vi "Read Dates.vi"(7 "SN":T2, 8 "error in (no error)":errorcluster, 9 "Calibration ID":T1, 10 "Time Stamp in":T3 {"Chamber Temp" format="%<%x>T"; "Probe 2 Temp" format="%<%x>T"; "Probe 1 Temp" format="%<%x>T"; "TC Panel 2" format="%<%x>T"; "TC Panel 1" format="%<%x>T"; "NI DAQ Card 7" format="%<%x>T"; "NI DAQ Card 6" format="%<%x>T"; "NI DAQ Card 5" format="%<%x>T"; "NI DAQ Card 4" format="%<%x>T"; "NI DAQ Card 3" format="%<%x>T"; "NI DAQ Card 2" format="%<%x>T"; "NI DAQ Card 1" format="%<%x>T"; "Gas Meter Thermocouple" format="%<%x>T"; "Gas Meter Pressure Transducer" format="%<%x>T"; "Gas Meter" format="%<%x>T"; "Sentra Scale" format="%<%x>T"; "B-Tech Scale" format="%<%x>T"; "Barometer" format="%<%x>T"; "WT 500" format="%<%x>T"; "Chroma" format="%<%x>T"}, 11 "file path (dialog if empty)":path) -> (0 "error out":errorcluster, 1 "SN.":T2, 2 "Calibration ID.":T1, 3 "Time Stamp out":T3 {"Chamber Temp" format="%<%x>T"; "Probe 2 Temp" format="%<%x>T"; "Probe 1 Temp" format="%<%x>T"; "TC Panel 2" format="%<%x>T"; "TC Panel 1" format="%<%x>T"; "NI DAQ Card 7" format="%<%x>T"; "NI DAQ Card 6" format="%<%x>T"; "NI DAQ Card 5" format="%<%x>T"; "NI DAQ Card 4" format="%<%x>T"; "NI DAQ Card 3" format="%<%x>T"; "NI DAQ Card 2" format="%<%x>T"; "NI DAQ Card 1" format="%<%x>T"; "Gas Meter Thermocouple" format="%<%x>T"; "Gas Meter Pressure Transducer" format="%<%x>T"; "Gas Meter" format="%<%x>T"; "Sentra Scale" format="%<%x>T"; "B-Tech Scale" format="%<%x>T"; "Barometer" format="%<%x>T"; "WT 500" format="%<%x>T"; "Chroma" format="%<%x>T"}, 4 "Size":i32, 5 "new file path (Not A Path if cancelled)":path)   [LabVIEW 2014]
uses:
  Type Definitions/CalibrationTime.ctl
  Type Definitions/Calibration.ctl
  Type Definitions/Calibration_SN.ctl
  <vilib>/Utility/file.llb/Read From Spreadsheet File (string).vi
panel:
  out "all rows":string[][](array[string])
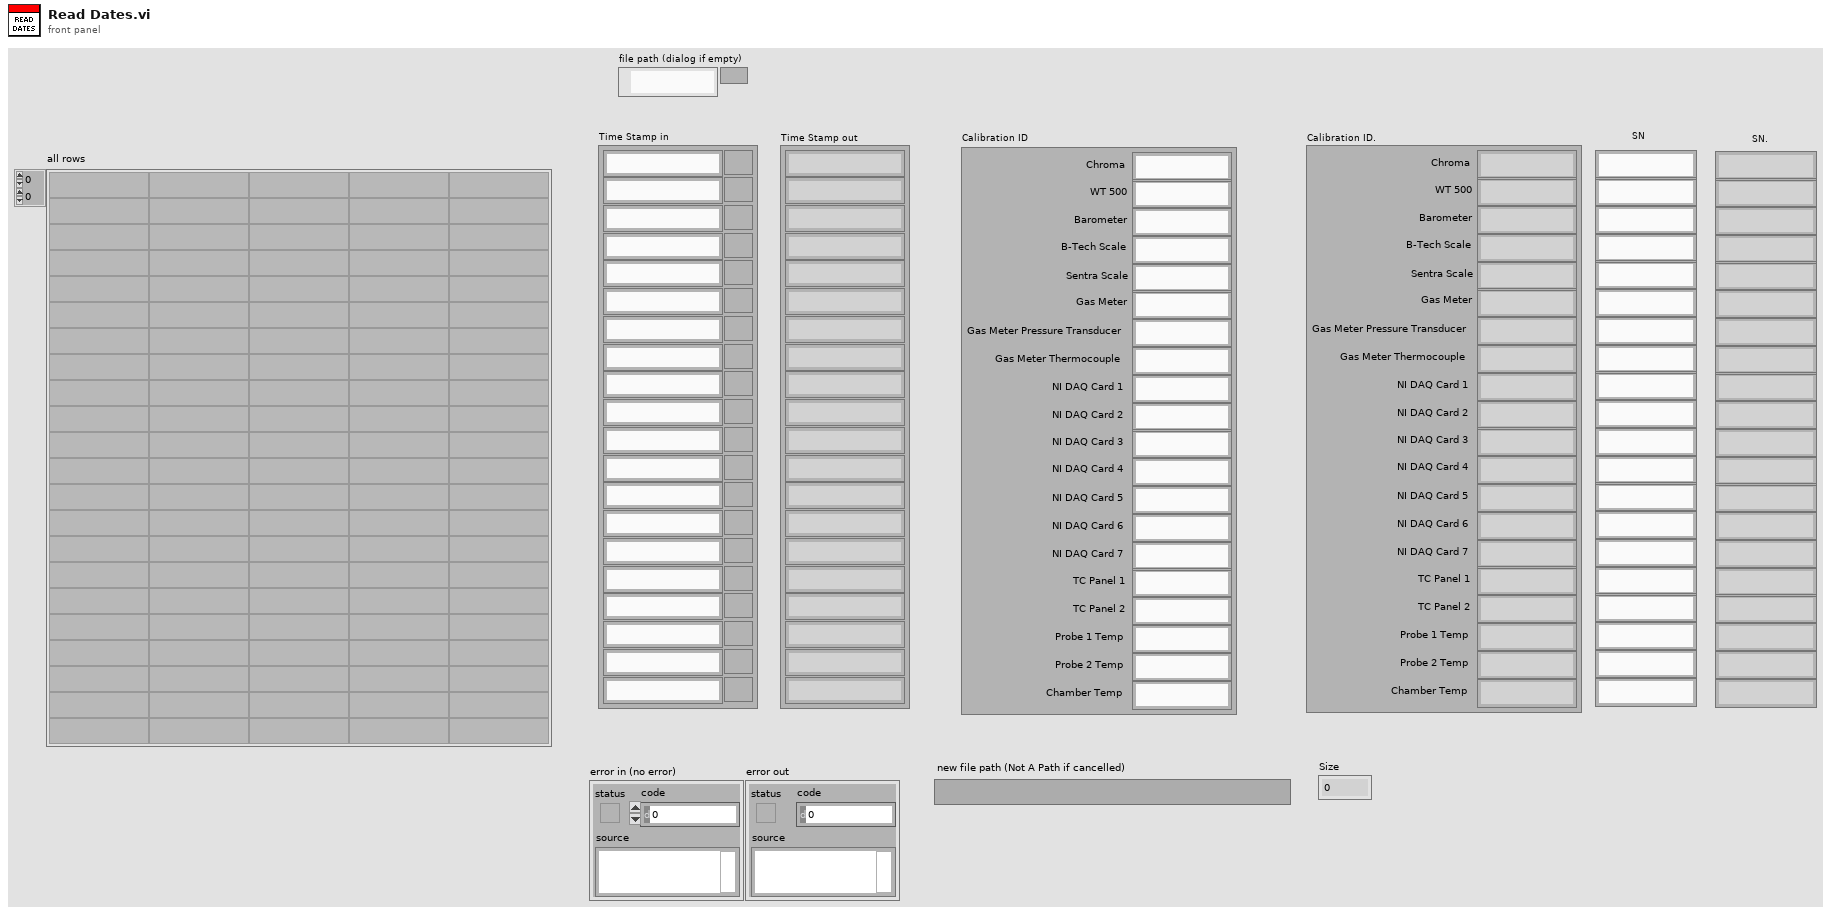
[diagram p1: front panel]
types:
  T1 = typedef "Calibration.ctl" = cluster{"Chroma":string, "WT 500":string, "Barometer":string, "B-Tech Scale":string, "Sentra Scale":string, "Gas Meter":string, "Gas Meter Pressure Transducer":string, "Gas Meter Thermocouple":string, "NI DAQ Card 1":string, "NI DAQ Card 2":string, "NI DAQ Card 3":string, "NI DAQ Card 4":string, "NI DAQ Card 5":string, "NI DAQ Card 6":string, "NI DAQ Card 7":string, "TC Panel 1":string, "TC Panel 2":string, "Probe 1 Temp":string, "Probe 2 Temp":string, "Chamber Temp":string}
  T2 = typedef "Calibration_SN.ctl" = cluster{"Chroma":string, "WT 500":string, "Barometer":string, "B-Tech Scale":string, "Sentra Scale":string, "Gas Meter":string, "Gas Meter Pressure Transducer":string, "Gas Meter Thermocouple":string, "NI DAQ Card 1":string, "NI DAQ Card 2":string, "NI DAQ Card 3":string, "NI DAQ Card 4":string, "NI DAQ Card 5":string, "NI DAQ Card 6":string, "NI DAQ Card 7":string, "TC Panel 1":string, "TC Panel 2":string, "Probe 1 Temp":string, "Probe 2 Temp":string, "Chamber Temp":string}
  T3 = typedef "CalibrationTime.ctl" = cluster{"Chroma":timestamp, "WT 500":timestamp, "Barometer":timestamp, "B-Tech Scale":timestamp, "Sentra Scale":timestamp, "Gas Meter":timestamp, "Gas Meter Pressure Transducer":timestamp, "Gas Meter Thermocouple":timestamp, "NI DAQ Card 1":timestamp, "NI DAQ Card 2":timestamp, "NI DAQ Card 3":timestamp, "NI DAQ Card 4":timestamp, "NI DAQ Card 5":timestamp, "NI DAQ Card 6":timestamp, "NI DAQ Card 7":timestamp, "TC Panel 1":timestamp, "TC Panel 2":timestamp, "Probe 1 Temp":timestamp, "Probe 2 Temp":timestamp, "Chamber Temp":timestamp}
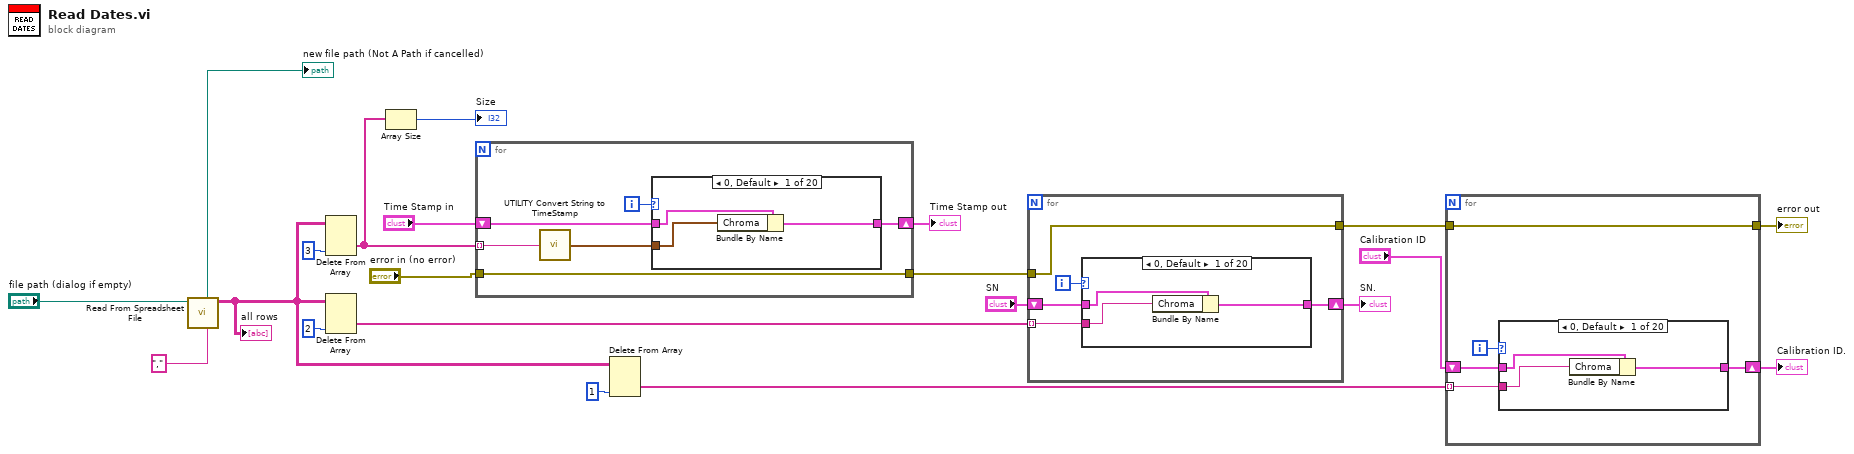
[diagram p0: block diagram]
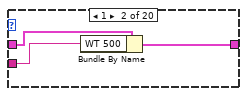
[diagram p2: hidden frame]
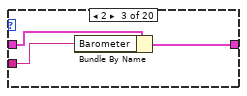
[diagram p3: hidden frame]
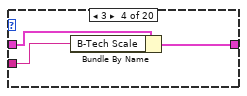
[diagram p4: hidden frame]
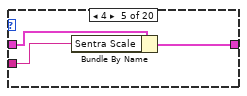
[diagram p5: hidden frame]
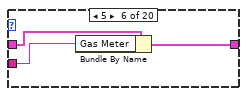
[diagram p6: hidden frame]
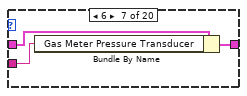
[diagram p7: hidden frame]
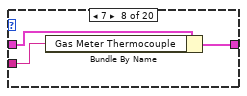
[diagram p8: hidden frame]
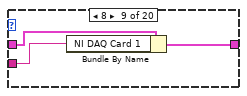
[diagram p9: hidden frame]
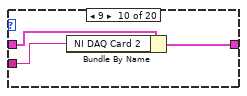
[diagram p10: hidden frame]
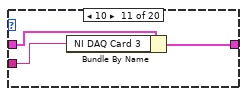
[diagram p11: hidden frame]
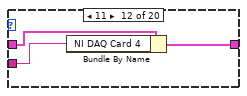
[diagram p12: hidden frame]
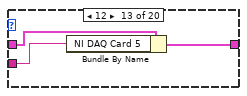
[diagram p13: hidden frame]
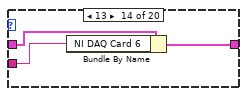
[diagram p14: hidden frame]
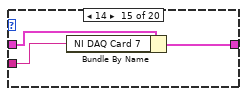
[diagram p15: hidden frame]
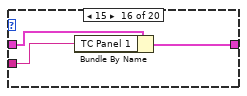
[diagram p16: hidden frame]
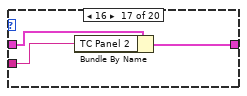
[diagram p17: hidden frame]
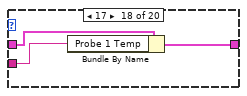
[diagram p18: hidden frame]
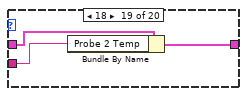
[diagram p19: hidden frame]
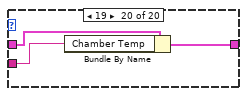
[diagram p20: hidden frame]
diagram:
  n1 = call-poly <vilib>:"Read From Spreadsheet File.vi"("delimiter (\\t)"="," ("delimiter (\\t)"), "file path (dialog if empty)"="file path (dialog if empty)") -> ("all rows"=w11:string[][], "new file path (Not A Path if cancelled)"=→"new file path (Not A Path if cancelled)":path)  [unwired: 5 in, 3 out]
  "all rows" <- w11
  n2 = Delete From Array(array=w11, index (col)=3 ("disabled index (col)")) -> (deleted portion=w2:string[])  [unwired: 2 in, 1 out]
  n3 = Delete From Array(array=w11, index (col)=2 ("disabled index (col)")) -> (deleted portion=w8:string[])  [unwired: 2 in, 1 out]
  n4 = Array Size(array=w2) -> (size(s)=→"Size":i32)
  n5 = for {
    tunnel: w2 -> [w27] mode=indexing
    shift-right: [w23] -> w18
    shift-left: "Time Stamp in" -> [w25]
    tunnel: [w22] -> w15
    tunnel: "error in (no error)" -> [w22]
    i -> [w26]
    n6 = call "UTILITY Convert String to TimeStamp.vi"("date/time string"=w27) -> ("Resulting Time Stamp"=w24:timestamp)
    n7 = case shown="0, Default" w26 {
      tunnel: w25 -> [w29 w32 w35 w38 w41 w44 w47 w50 w53 w56 w59 w62 w65 w68 w72 w75 w78 w81 w83 w86]
      tunnel: w24 -> [w30 w33 w36 w39 w42 w45 w48 w51 w54 w57 w60 w63 w66 w69 w71 w74 w77 w79 w84 w87]
      tunnel: [w28 w31 w34 w37 w40 w43 w46 w49 w52 w55 w58 w61 w64 w67 w70 w73 w76 w80 w82 w85] -> w23
      frame 0, Default {
        n8 = Bundle By Name(cluster=w29, "Chroma"=w30) -> (w28:T3)
      }
      frame 1 {
        n9 = Bundle By Name(cluster=w32, "WT 500"=w33) -> (w31:T3)
      }
      frame 2 {
        n10 = Bundle By Name(cluster=w35, "Barometer"=w36) -> (w34:T3)
      }
      frame 3 {
        n11 = Bundle By Name(cluster=w38, "B-Tech Scale"=w39) -> (w37:T3)
      }
      frame 4 {
        n12 = Bundle By Name(cluster=w41, "Sentra Scale"=w42) -> (w40:T3)
      }
      frame 5 {
        n13 = Bundle By Name(cluster=w44, "Gas Meter"=w45) -> (w43:T3)
      }
      frame 6 {
        n14 = Bundle By Name(cluster=w47, "Gas Meter Pressure Transducer"=w48) -> (w46:T3)
      }
      frame 7 {
        n15 = Bundle By Name(cluster=w50, "Gas Meter Thermocouple"=w51) -> (w49:T3)
      }
      frame 8 {
        n16 = Bundle By Name(cluster=w53, "NI DAQ Card 1"=w54) -> (w52:T3)
      }
      frame 9 {
        n17 = Bundle By Name(cluster=w56, "NI DAQ Card 2"=w57) -> (w55:T3)
      }
      frame 10 {
        n18 = Bundle By Name(cluster=w59, "NI DAQ Card 3"=w60) -> (w58:T3)
      }
      frame 11 {
        n19 = Bundle By Name(cluster=w62, "NI DAQ Card 4"=w63) -> (w61:T3)
      }
      frame 12 {
        n20 = Bundle By Name(cluster=w65, "NI DAQ Card 5"=w66) -> (w64:T3)
      }
      frame 13 {
        n21 = Bundle By Name(cluster=w68, "NI DAQ Card 6"=w69) -> (w67:T3)
      }
      frame 14 {
        n22 = Bundle By Name(cluster=w72, "NI DAQ Card 7"=w71) -> (w70:T3)
      }
      frame 15 {
        n23 = Bundle By Name(cluster=w75, "TC Panel 1"=w74) -> (w73:T3)
      }
      frame 16 {
        n24 = Bundle By Name(cluster=w78, "TC Panel 2"=w77) -> (w76:T3)
      }
      frame 17 {
        n25 = Bundle By Name(cluster=w81, "Probe 1 Temp"=w79) -> (w80:T3)
      }
      frame 18 {
        n26 = Bundle By Name(cluster=w83, "Probe 2 Temp"=w84) -> (w82:T3)
      }
      frame 19 {
        n27 = Bundle By Name(cluster=w86, "Chamber Temp"=w87) -> (w85:T3)
      }
    }
  }
  "Time Stamp out" <- w18
  n28 = Delete From Array(array=w11, index (col)=1 ("disabled index (col)")) -> (deleted portion=w7:string[])  [unwired: 2 in, 1 out]
  n29 = for {
    tunnel: w8 -> [w88] mode=indexing
    shift-right: [w90] -> w4
    shift-left: "SN" -> [w91]
    tunnel: [w89] -> w14
    tunnel: w15 -> [w89]
    i -> [w92]
    n30 = case shown="0, Default" w92 {
      tunnel: w91 -> [w95 w98 w101 w104 w107 w110 w113 w116 w119 w122 w125 w128 w131 w134 w137 w140 w142 w145 w148 w151]
      tunnel: [w94 w97 w100 w103 w106 w109 w112 w115 w118 w121 w124 w127 w130 w133 w136 w138 w141 w144 w147 w150] -> w90
      tunnel: w88 -> [w93 w96 w99 w102 w105 w108 w111 w114 w117 w120 w123 w126 w129 w132 w135 w139 w143 w146 w149 w152]
      frame 0, Default {
        n31 = Bundle By Name(cluster=w95, "Chroma"=w93) -> (w94:T2)
      }
      frame 1 {
        n32 = Bundle By Name(cluster=w98, "WT 500"=w96) -> (w97:T2)
      }
      frame 2 {
        n33 = Bundle By Name(cluster=w101, "Barometer"=w99) -> (w100:T2)
      }
      frame 3 {
        n34 = Bundle By Name(cluster=w104, "B-Tech Scale"=w102) -> (w103:T2)
      }
      frame 4 {
        n35 = Bundle By Name(cluster=w107, "Sentra Scale"=w105) -> (w106:T2)
      }
      frame 5 {
        n36 = Bundle By Name(cluster=w110, "Gas Meter"=w108) -> (w109:T2)
      }
      frame 6 {
        n37 = Bundle By Name(cluster=w113, "Gas Meter Pressure Transducer"=w111) -> (w112:T2)
      }
      frame 7 {
        n38 = Bundle By Name(cluster=w116, "Gas Meter Thermocouple"=w114) -> (w115:T2)
      }
      frame 8 {
        n39 = Bundle By Name(cluster=w119, "NI DAQ Card 1"=w117) -> (w118:T2)
      }
      frame 9 {
        n40 = Bundle By Name(cluster=w122, "NI DAQ Card 2"=w120) -> (w121:T2)
      }
      frame 10 {
        n41 = Bundle By Name(cluster=w125, "NI DAQ Card 3"=w123) -> (w124:T2)
      }
      frame 11 {
        n42 = Bundle By Name(cluster=w128, "NI DAQ Card 4"=w126) -> (w127:T2)
      }
      frame 12 {
        n43 = Bundle By Name(cluster=w131, "NI DAQ Card 5"=w129) -> (w130:T2)
      }
      frame 13 {
        n44 = Bundle By Name(cluster=w134, "NI DAQ Card 6"=w132) -> (w133:T2)
      }
      frame 14 {
        n45 = Bundle By Name(cluster=w137, "NI DAQ Card 7"=w135) -> (w136:T2)
      }
      frame 15 {
        n46 = Bundle By Name(cluster=w140, "TC Panel 1"=w139) -> (w138:T2)
      }
      frame 16 {
        n47 = Bundle By Name(cluster=w142, "TC Panel 2"=w143) -> (w141:T2)
      }
      frame 17 {
        n48 = Bundle By Name(cluster=w145, "Probe 1 Temp"=w146) -> (w144:T2)
      }
      frame 18 {
        n49 = Bundle By Name(cluster=w148, "Probe 2 Temp"=w149) -> (w147:T2)
      }
      frame 19 {
        n50 = Bundle By Name(cluster=w151, "Chamber Temp"=w152) -> (w150:T2)
      }
    }
  }
  "SN." <- w4
  n51 = for {
    tunnel: w7 -> [w153] mode=indexing
    shift-right: [w155] -> w3
    shift-left: "Calibration ID" -> [w156]
    tunnel: [w154] -> w13
    tunnel: w14 -> [w154]
    i -> [w157]
    n52 = case shown="0, Default" w157 {
      tunnel: w156 -> [w159 w162 w165 w168 w171 w174 w177 w180 w183 w186 w189 w192 w195 w198 w202 w204 w207 w210 w213 w216]
      tunnel: w153 -> [w160 w163 w166 w169 w172 w175 w178 w181 w184 w187 w190 w193 w196 w199 w201 w205 w208 w211 w214 w217]
      tunnel: [w158 w161 w164 w167 w170 w173 w176 w179 w182 w185 w188 w191 w194 w197 w200 w203 w206 w209 w212 w215] -> w155
      frame 0, Default {
        n53 = Bundle By Name(cluster=w159, "Chroma"=w160) -> (w158:T1)
      }
      frame 1 {
        n54 = Bundle By Name(cluster=w162, "WT 500"=w163) -> (w161:T1)
      }
      frame 2 {
        n55 = Bundle By Name(cluster=w165, "Barometer"=w166) -> (w164:T1)
      }
      frame 3 {
        n56 = Bundle By Name(cluster=w168, "B-Tech Scale"=w169) -> (w167:T1)
      }
      frame 4 {
        n57 = Bundle By Name(cluster=w171, "Sentra Scale"=w172) -> (w170:T1)
      }
      frame 5 {
        n58 = Bundle By Name(cluster=w174, "Gas Meter"=w175) -> (w173:T1)
      }
      frame 6 {
        n59 = Bundle By Name(cluster=w177, "Gas Meter Pressure Transducer"=w178) -> (w176:T1)
      }
      frame 7 {
        n60 = Bundle By Name(cluster=w180, "Gas Meter Thermocouple"=w181) -> (w179:T1)
      }
      frame 8 {
        n61 = Bundle By Name(cluster=w183, "NI DAQ Card 1"=w184) -> (w182:T1)
      }
      frame 9 {
        n62 = Bundle By Name(cluster=w186, "NI DAQ Card 2"=w187) -> (w185:T1)
      }
      frame 10 {
        n63 = Bundle By Name(cluster=w189, "NI DAQ Card 3"=w190) -> (w188:T1)
      }
      frame 11 {
        n64 = Bundle By Name(cluster=w192, "NI DAQ Card 4"=w193) -> (w191:T1)
      }
      frame 12 {
        n65 = Bundle By Name(cluster=w195, "NI DAQ Card 5"=w196) -> (w194:T1)
      }
      frame 13 {
        n66 = Bundle By Name(cluster=w198, "NI DAQ Card 6"=w199) -> (w197:T1)
      }
      frame 14 {
        n67 = Bundle By Name(cluster=w202, "NI DAQ Card 7"=w201) -> (w200:T1)
      }
      frame 15 {
        n68 = Bundle By Name(cluster=w204, "TC Panel 1"=w205) -> (w203:T1)
      }
      frame 16 {
        n69 = Bundle By Name(cluster=w207, "TC Panel 2"=w208) -> (w206:T1)
      }
      frame 17 {
        n70 = Bundle By Name(cluster=w210, "Probe 1 Temp"=w211) -> (w209:T1)
      }
      frame 18 {
        n71 = Bundle By Name(cluster=w213, "Probe 2 Temp"=w214) -> (w212:T1)
      }
      frame 19 {
        n72 = Bundle By Name(cluster=w216, "Chamber Temp"=w217) -> (w215:T1)
      }
    }
  }
  "error out" <- w13
  "Calibration ID." <- w3
